vi "FP Find red target.vi"(0 "Image In":T1, 1 "error in (no error)":errorcluster) -> (2 "Image Dst Out":T1, 3 "Nb Circles (Circle Detection 1)":i32, 4 "Camera Data":T2(array[cluster]), 5 "error out":errorcluster)   [LabVIEW 2014]
doc: "This VI takes in an image and finds a round, red target. It produces the target location and size."
uses:
  <vilib>/vision/Image Controls.llb/IMAQ Image.ctl
  <vilib>/vision/NI_Vision_Development_Module.lvlib
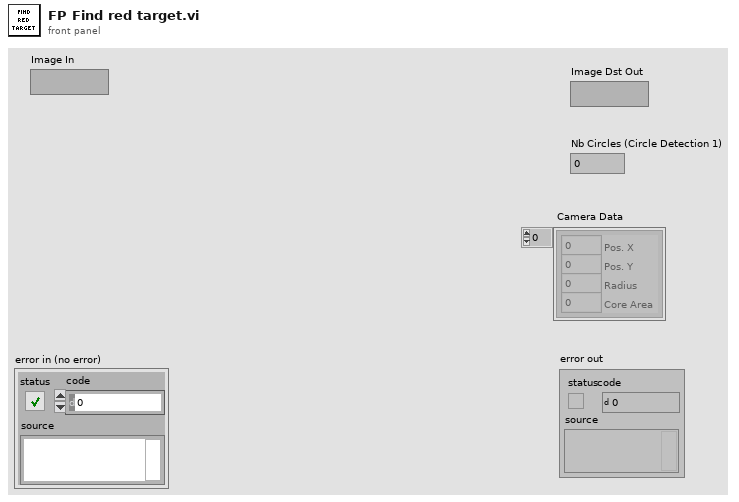
[diagram p1: front panel]
types:
  T1 = typedef "IMAQ Image.ctl" = refnum<image>
  T2 = cluster{"Pos. X":i32, "Pos. Y":i32, "Radius":i32, "Core Area":i32}[]
  T3 = enum32{"AutoM", "Close", "Dilate", "Erode", "Gradient", "Gradient in", "Gradient out", "HitMiss", "Open", "PClose", "POpen", "Thick", "Thin"}
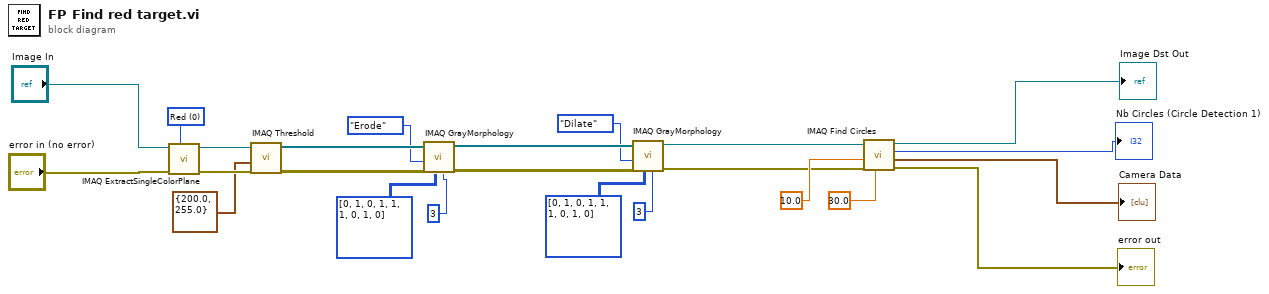
[diagram p0: block diagram]
diagram:
  w24 = 0 items=["Red", "Green", "Blue", "Hue", "Saturation", "Luminance", "Value", "Intensity"] ("Color Plane (Color Plane Extraction 1)")
  n1 = call "IMAQ ExtractSingleColorPlane"("Color Plane"=w24, "error in (no error)"="error in (no error)", "Image Src"="Image In") -> ("error out"=w22:errorcluster, "Image Dst Out"=w20:T1)  [unwired: 1 in, 6 out]
  n2 = call "IMAQ Threshold"("error in (no error)"=w22, "Range"=cluster{"Lower value":sgl, "Upper value":sgl} {"Lower value"=200.0, "Upper value"=255.0}, "Image Src"=w20) -> ("error out"=w19:errorcluster, "Image Dst Out"=w16:T1)  [unwired: 3 in, 4 out]
  n3 = call "IMAQ GrayMorphology"("Number of iterations (1)"=3 ("Number of iterations (1) (Gray Morphology 1)"), "Structuring Element"=i32[][] [[0, 1, 0], [1, 1, 1], [0, 1, 0]], "error in (no error)"=w19, "Operation"=T3."Erode" ("Operation (Gray Morphology 1)"), "Image Src"=w16) -> ("error out"=w15:errorcluster, "Image Dst Out"=w11:T1)  [unwired: 2 in, 3 out]
  n4 = call "IMAQ GrayMorphology"("Number of iterations (1)"=3 ("Number of iterations (1) (Gray Morphology 2)"), "Structuring Element"=i32[][] [[0, 1, 0], [1, 1, 1], [0, 1, 0]], "error in (no error)"=w15, "Operation"=T3."Dilate" ("Operation (Gray Morphology 2)"), "Image Src"=w11) -> ("error out"=w4:errorcluster, "Image Dst Out"=w6:T1)  [unwired: 2 in, 3 out]
  n5 = call "IMAQ Find Circles"("Max Radius"=sgl 30.0 ("Max Radius (Circle Detection 1)"), "error in (no error)"=w4, "Min Radius"=sgl 10.0 ("Min Radius (Circle Detection 1)"), "Image Src"=w6) -> ("error out"=→"error out":errorcluster, "Circles Data"=→"Camera Data":T2, "Nb Circles"=→"Nb Circles (Circle Detection 1)":i32, "Image Dst Out"=→"Image Dst Out":T1)  [unwired: 1 in, 3 out]
